vi "Append Control Image to Report.vi"(0 "report in":refnum<class "NI_HTML.lvclass">, 1 "alignment (default)":T2, 2 "image file type (.jpg)":enum16{".jpg", ".png"}(ring), 5 "image depth":T1=2 items=["B&W", "4 bits", "8 bits", "24 bits"], 7 "ctrl reference":refnum<vi>, 9 "description":string, 11 "error in (no error)":errorcluster, 12 "MS Office parameters":T3) -> (4 "report out":refnum<class "NI_HTML.lvclass">, 8 "start out (Word)":i32, 10 "end out (Word)":i32, 15 "error out":errorcluster)   [LabVIEW 2017, in "NI_HTML.lvclass"]
doc: "Creates an image of the front panel object specified in <B>Ctrl Reference</B> and appends it to a report."
uses:
  <vilib>/Utility/NIReport.llb/HTML/NI_HTML.lvclass
  <vilib>/Utility/NIReport.llb/HTML Report Image Alignment.ctl
  <vilib>/Utility/NIReport.llb/image depth.ctl
  <vilib>/Utility/NIReport.llb/HTML/NI_HTML.lvclass/NI_HTML.ctl
  <vilib>/Utility/NIReport.llb/NI_ReportGenerationCore.lvlib
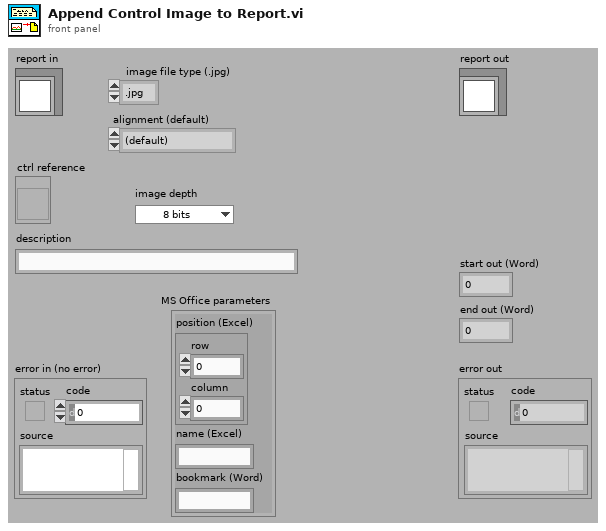
[diagram p1: front panel]
types:
  T1 = typedef "NI_ReportGenerationCore.lvlib/image depth.ctl" = u16
  T2 = typedef "NI_ReportGenerationCore.lvlib/HTML Report Image Alignment.ctl" = enum16{"(default)", "LEFT", "RIGHT", "TOP", "TEXTTOP", "MIDDLE", "ABSMIDDLE", "BASELINE", "BOTTOM", "ABSBOTTOM"}
  T3 = cluster{"position (Excel)":cluster{"row":i32, "column":i32}, "name (Excel)":string, "bookmark (Word)":string}
  T4 = typedef "NI_ReportGenerationCore.lvlib/HTML Report Data.ctl" = cluster{"Body Text":string, "Font Tag":string, "Title Text":string, "Header Text":string, "Footer Text":string, "Image List":path[]}
  T5 = typedef "imagedata.ctl" = cluster{"image type":i32, "image depth":i32, "image":u8[], "mask":u8[], "colors":u32[], "Rectangle":cluster{"left":i16, "top":i16, "right":i16, "bottom":i16}}
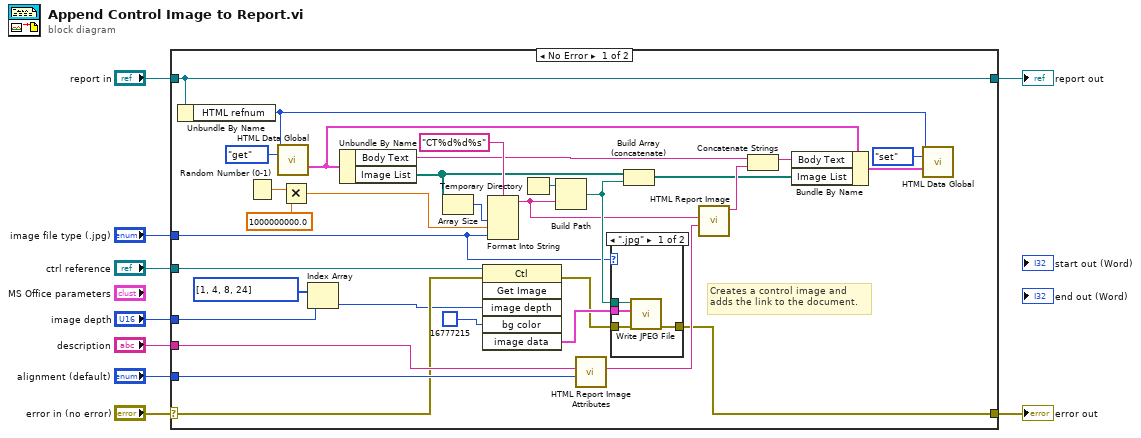
[diagram p0: block diagram]
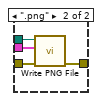
[diagram p2: hidden frame]
diagram:
  n1 = case shown="No Error" "error in (no error)" {
    selector: "error in (no error)" -> [w27 w51]
    tunnel: [w26 w51] -> w8
    tunnel: [w21 w50] -> w6
    tunnel: "report in" -> [w21 w50]
    tunnel: "ctrl reference" -> [w31 _]
    tunnel: "image file type (.jpg)" -> [w30 _]
    tunnel: "description" -> [w29 _]
    tunnel: "alignment (default)" -> [w28 _]
    tunnel: "image depth" -> [w14 _]
    frame No Error {
      # "Creates a control image and\nadds the link to the document."
      n2 = Unbundle By Name(w21) -> ("HTML refnum"=w16:u32)
      n3 = Random Number (0-1)() -> (number: 0 to 1=w12:dbl)
      n4 = call <vilib>:"HTML Data Global.vi"("HTML refnum"=w16, "menu"=enum16{"init", "get", "set", "delete"}."get") -> ("HTML report data out"=w20:T4)  [unwired: 1 in, 12 out]
      n5 = Multiply(x=w12, y=1000000000.0) -> (x*y=w10:dbl)
      n6 = Index Array(array=i32[] [1, 4, 8, 24] ("Array Constant"), index=w14) -> (element=w13:i32)
      n7 = Unbundle By Name(w20) -> ("Body Text"=w22:string, "Image List"=w25:path[])
      n8 = Array Size(array=w25) -> (size(s)=w34:i32)
      n9 = invoke class="Ctl" method="Get Image"(reference=w31, error in=w27, "image depth"=w13, "bg color"=u32 16777215) -> (error out=w39:errorcluster, "image data"=w41:T5)  [unwired: 2 in, 4 out]
      n10 = Format Into String(format string="CT%d%d%s" ("Format String"), w34, w10, w30) -> (resulting string=w36:string)  [unwired: 2 in, 1 out]
      n11 = Temporary Directory() -> (w33:path)
      n12 = Build Path(base path=w33, name or relative path=w36) -> (appended path=w40:path)
      n13 = call <vilib>:"HTML Report Image Attributes.vi"("alignment (default)"=w28, "alt - alternative string"=w29) -> ("attributes out"=w37:string)  [unwired: 5 out]
      n14 = case shown="\".jpg\"" w30 {
        tunnel: w39 -> [w43 w48]
        tunnel: [w42 w49] -> w26
        tunnel: w40 -> [w45 w46]
        tunnel: w41 -> [w44 w47]
        frame ".jpg" {
          n15 = call <vilib>:"Write JPEG File.vi"("error in (no error)"=w43, "image data"=w44, "path to JPEG file"=w45) -> ("error out"=w42:errorcluster)  [unwired: 8 out]
        }
        frame ".png" {
          n16 = call <vilib>:"Write PNG File.vi"("error in (no error)"=w48, "image data"=w47, "path to PNG file"=w46) -> ("error out"=w49:errorcluster)  [unwired: 8 out]
        }
      }
      n17 = Build Array (concatenate)(w25, w40) -> (w24:path[])
      n18 = call <vilib>:"HTML Report Image.vi"("image attributes"=w37, "src - URL of image to embed"=w36) -> ("HTML out"=w32:string)  [unwired: 2 in, 7 out]
      n19 = Concatenate Strings(w22, w32) -> (w19:string)
      n20 = Bundle By Name(cluster=w20, "Body Text"=w19, "Image List"=w24) -> (w17:T4)
      n21 = call <vilib>:"HTML Data Global.vi"("HTML refnum"=w16, "menu"=enum16{"init", "get", "set", "delete"}."set", "HTML report data in"=w17) -> ()  [unwired: 13 out]
    }
    frame Error {
    }
  }
  "error out" <- w8
  "report out" <- w6
